vi "Delimited String to 1D Array.vi"(10 "Delimiter (,)":string=",", 11 "Delimited String":string) -> (3 "String Array":string[](array[string]))   [LabVIEW 2022 SP3, in "hse-misc.lvlib"]
doc: "Converts a delimited string (e.g. \"A, B, C\") to an 1D array of strings (e.g. [\"A\", \"B\", \"C\"]. Removes whitespace around the elements.\n\n____\nHAMPEL SOFTWARE ENGINEERING v3.8.0 (2023-12-18 14:41)"
uses:
  hse-misc.lvlib
  <vilib>/Utility/error.llb/Trim Whitespace One-Sided.vi
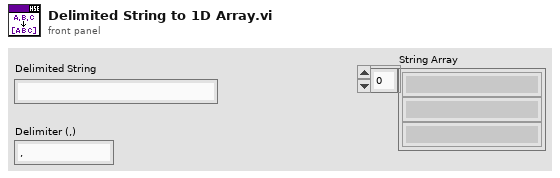
[diagram p1: front panel]
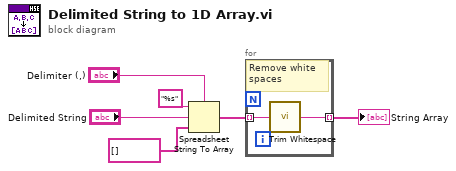
[diagram p0: block diagram]
diagram:
  n1 = Spreadsheet String To Array(delimiter (Tab)="Delimiter (,)", format string="%s", spreadsheet string="Delimited String", array type (2D Dbl)=string[] []) -> (array=w2:string[])
  n2 = for {
    tunnel: w2 -> [w8] mode=indexing
    tunnel: [w7] -> w1 mode=indexing
    # "Remove white spaces"
    n3 = call <vilib>:"Trim Whitespace.vi"("string"=w8) -> ("trimmed string"=w7:string)  [unwired: 1 in]
  }
  "String Array" <- w1
